vi "SetSpeed.vi"(8 "error in (no error)":errorcluster, 10 "RPM":u16, 11 "StepperMotor in":refnum<class "StepperMotor.lvclass">) -> (0 "error out":errorcluster, 3 "StepperMotor out":refnum<class "StepperMotor.lvclass">)   [LabVIEW 2022 SP3, in "Motorshield.lvlib" / "StepperMotor.lvclass"]
uses:
  StepperMotor.lvclass
  StepperMotor.lvclass/StepperMotor.ctl
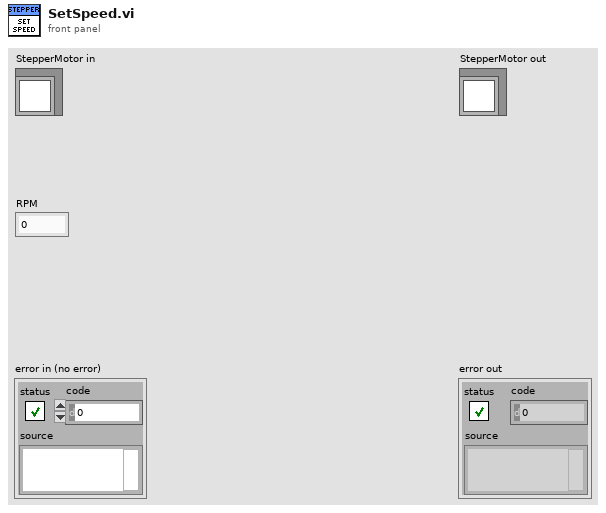
[diagram p1: front panel]
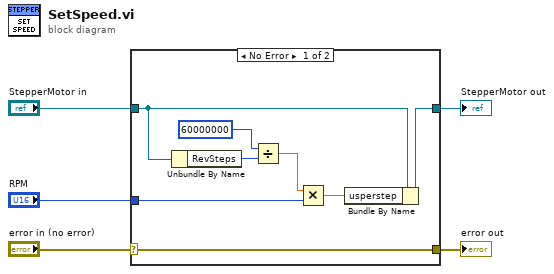
[diagram p0: block diagram]
diagram:
  n1 = case shown="No Error" "error in (no error)" {
    selector: "error in (no error)" -> [w13 w15]
    tunnel: [w13 w15] -> w4
    tunnel: [w12 w14] -> w2
    tunnel: "StepperMotor in" -> [w10 w14]
    tunnel: "RPM" -> [w8 _]
    frame No Error {
      n2 = Unbundle By Name(w10) -> ("RevSteps"=w9:u16)
      n3 = Divide(x=60000000, y=w9) -> (x/y=w7:dbl)
      n4 = Multiply(x=w7, y=w8) -> (x*y=w6:dbl)
      n5 = Bundle By Name(cluster=w10, "usperstep"=w6) -> (w12:refnum<class "StepperMotor.lvclass">)
    }
    frame Error {
    }
  }
  "error out" <- w4
  "StepperMotor out" <- w2
